vi "Angles_flt.vi"() -> (1 "psi":dbl, 2 "phi":dbl, 3 "theta":dbl)   [LabVIEW 2017]
uses:
  <userlib>/HapticSTM/HapticSTM.lvlib
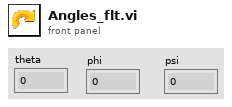
[diagram p1: front panel]
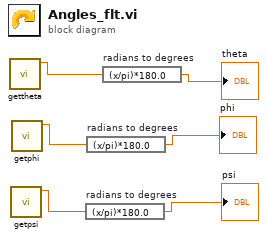
[diagram p0: block diagram]
diagram:
  n1 = call <userlib>:"gettheta.vi"() -> ("function return"=w6:dbl)  [unwired: 11 in]
  n2 = call <userlib>:"getpsi.vi"() -> ("function return"=w2:dbl)  [unwired: 11 in]
  n3 = call <userlib>:"getphi.vi"() -> ("function return"=w4:dbl)  [unwired: 11 in]
  n4 = expression code="(x/pi)*180.0" "radians to degrees"(w2) -> (→"psi":dbl)
  n5 = expression code="(x/pi)*180.0" "radians to degrees"(w4) -> (→"phi":dbl)
  n6 = expression code="(x/pi)*180.0" "radians to degrees"(w6) -> (→"theta":dbl)
